vi "Memory.Pointer.Clear.vi"(8 "error in (no error)":errorcluster, 11 "pointer in":refnum<class "Memory.Pointer.lvclass">) -> (0 "error out":errorcluster, 3 "pointer out":refnum<class "Memory.Pointer.lvclass">)   [LabVIEW 2016, in "Memory Manager.lvlib" / "Memory.Pointer.lvclass"]
doc: "Sets the bytes specified by <b>pointer</b> to zero."
uses:
  Memory.Pointer.lvclass
  Memory.Pointer.lvclass/Memory.Pointer.ctl
  Memory.Pointer.Errors.vi
  Memory.Pointer.Errors.Null Pointer.vi
  Memory.Pointer.Errors.Create Error.vi
  Submodules/SEH/Source/VIs/Static Error Handling.Error Cluster Constant.vi
  Submodules/SEH/Source/VIs/Static Error Handling.Error Cluster Constant (256B).vi
  Submodules/SEH/Source/VIs/Static Error Handling.Parameters.Status.Set.vi
  Submodules/SEH/Source/VIs/Static Error Handling.Parameters.Code.Set.vi
  Submodules/SEH/Source/VIs/Static Error Handling.Parameters.VI Source.Set.vi
  Constants/Memory.Constants.vi
  Constants/Memory.Constants.Library Name.vi
  Memory.Pointer.Errors.Get Info.vi
  Submodules/SEH/Source/VIs/Static Error Handling.Source Buffer.Write.String.vi
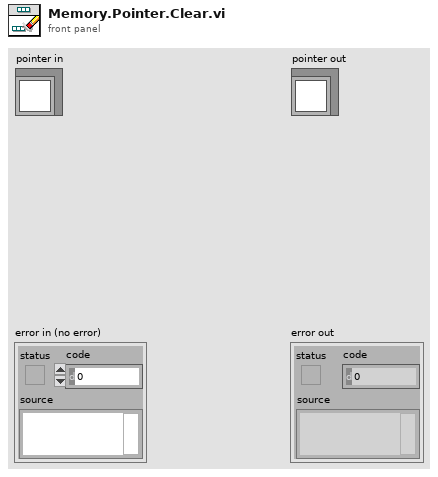
[diagram p1: front panel]
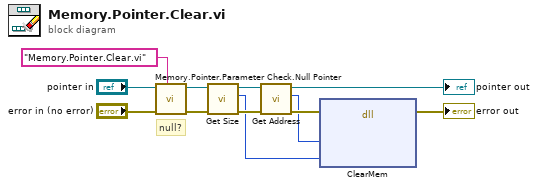
[diagram p0: block diagram]
diagram:
  # "null?"
  n1 = call "Memory.Pointer.Parameter Check.Null Pointer.vi"("source vi name"="Memory.Pointer.Clear.vi", "error in (no error)"="error in (no error)", "Pointer in"="pointer in") -> ("error out"=w2:errorcluster, "Pointer out"=w3:refnum<class "Memory.Pointer.lvclass">)  [unwired: 7 in]
  n2 = call "Get Size.vi"("error in (no error)"=w2, "Pointer in"=w3) -> ("error out"=w9:errorcluster, "size"=w7:u64, "Pointer out"=w12:refnum<class "Memory.Pointer.lvclass">)  [unwired: 7 in]
  n3 = call "Get Address.vi"("error in (no error)"=w9, "Pointer in"=w12) -> ("error out"=w11:errorcluster, "address"=w6:u64, "Pointer out"=→"pointer out":refnum<class "Memory.Pointer.lvclass">)  [unwired: 7 in]
  n4 = dll-call lib="LabVIEW" fn="ClearMem"(error in=w11, "pointer"=w6, "size"=w7) -> (error out=→"error out":errorcluster)  [unwired: 5 in, 1 out]
